vi "Unsubscribe.vi"(6 "Subscriber Name":string, 7 "Topic Name":string, 8 "error in (no error)":errorcluster, 11 "Message Broker in":refnum<class "Message Broker.lvclass">) -> (0 "error out":errorcluster, 3 "Message Broker out":refnum<class "Message Broker.lvclass">)   [LabVIEW 2016, in "Stream Mediator.lvlib" / "Message Broker.lvclass"]
doc: "--\nCopyright © 2017 Composed SystemsI All rights reserved.\n\nAuthor: Jon McBee <jon.mcbee@composed.io>\n\nThis library is provided \"AS IS\" ,WITHOUT WARRANTIES OR\nCONDITIONS OF ANY KIND, either express or implied.\n\nComposed Systems -- composed.io\n\nStream 0.0.1.1\nJon McBee - Composed Systems\nCopyright (c) 2017, Composed Systems"
uses:
  <userlib>/Composed Systems/Stream/Mediator/Classes/Message Broker/Message Broker.lvclass
  <userlib>/Composed Systems/Stream/Mediator/Classes/Message Broker/Message Broker.lvclass/Message Broker.ctl
  <userlib>/Composed Systems/Stream/Mediator/Classes/Topic Actor Unsubscribe Command/Topic Actor Unsubscribe Command.lvclass
  C:/Program Files (x86)/National Instruments/LabVIEW 2016/user.lib/Composed Systems/Stream/Mediator/Classes/Message Interface/Message Interface.lvclass
  <userlib>/Composed Systems/Stream/Mediator/Classes/Message Transport Queue/Message Transport Queue.lvclass
  <userlib>/Composed Systems/Stream/Mediator/Classes/Topic Actor Look Up Table/Topic Actor Look Up Table.lvclass
  <userlib>/Composed Systems/Stream/Mediator/Classes/Topic Actor Descriptor/Topic Actor Descriptor.lvclass
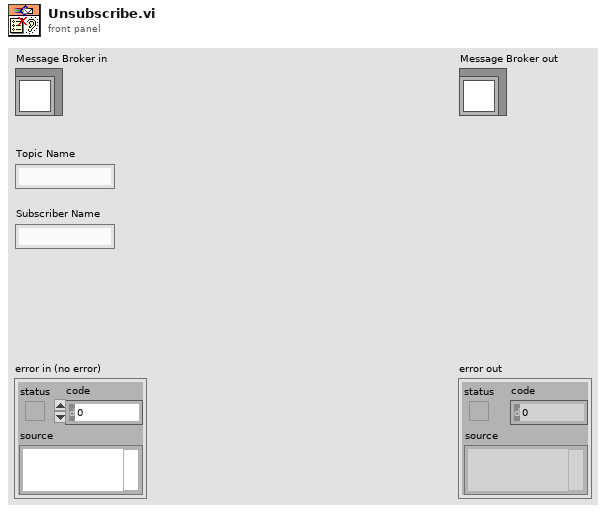
[diagram p1: front panel]
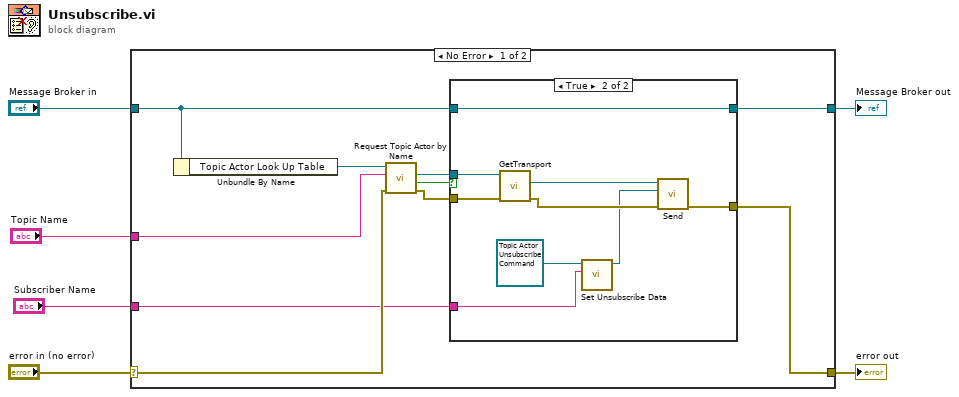
[diagram p0: block diagram]
diagram:
  n1 = case shown="No Error" "error in (no error)" {
    selector: "error in (no error)" -> [w10 w29]
    tunnel: [w9 w29] -> w5
    tunnel: [w14 w28] -> w3
    tunnel: "Message Broker in" -> [w15 w28]
    tunnel: "Topic Name" -> [w8 _]
    tunnel: "Subscriber Name" -> [w7 _]
    frame No Error {
      n2 = Unbundle By Name(w15) -> ("Topic Actor Look Up Table"=w16:refnum<class "Topic Actor Look Up Table.lvclass">)
      n3 = call <userlib>:"Request Topic Actor by Name.vi"("error in (no error)"=w10, "Topic Actor"=w8, "Topic Actor Look Up Table in"=w16) -> ("error out"=w11:errorcluster, "Found?"=w13:bool, "Topic Actor Descriptor"=w12:refnum<class "Topic Actor Descriptor.lvclass">)  [unwired: 5 in, 1 out]
      n4 = case shown="True" w13 {
        tunnel: [w18 w27] -> w14
        tunnel: w15 -> [w18 w27]
        tunnel: w12 -> [_ w26]
        tunnel: w11 -> [w17 w24]
        tunnel: [w17 w22] -> w9
        tunnel: w7 -> [_ w19]
        frame False {
        }
        frame True {
          n5 = call <userlib>:"GetTransport.vi"("error in (no error)"=w24, "Topic Actor Descriptor in"=w26) -> ("error out"=w23:errorcluster, "Transport"=w25:refnum<class "Message Transport Queue.lvclass">)  [unwired: 7 in, 1 out]
          n6 = call <userlib>:"Set Unsubscribe Data.vi"("Subscriber Name"=w19, "Topic Actor Unsubscribe Command in"=refnum<class "Topic Actor Unsubscribe Command.lvclass"> refnum ("Topic Actor Unsubscribe Command.lvclass")) -> ("Topic Actor Unsubscribe Command out"=w20:refnum<class "Topic Actor Unsubscribe Command.lvclass">)  [unwired: 8 in, 1 out]
          n7 = call-dynamic "Send.vi"("error in (no error)"=w23, "Message"=w20, "Message Transport Queue in"=w25) -> ("error out"=w22:errorcluster)  [unwired: 6 in, 2 out]
        }
      }
    }
    frame Error {
    }
  }
  "error out" <- w5
  "Message Broker out" <- w3
